vi "Polynomial Evaluation.vi"   [LabVIEW 2017, in "NI_AALPro.lvlib"]
doc: "Evaluates the polynomial <B>P(x)</B> with a single value or multiple values. The data types you wire to the <B>a</B> and <B>P(x)</B> inputs determine the polymorphic instance to use."
uses:
  <vilib>/Analysis/NI_AALPro.lvlib
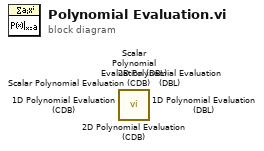
[diagram p0: block diagram]
diagram:
  n1 = call <vilib>:"2D Polynomial Evaluation (CDB).vi"() -> ()  [unwired: 2 in, 2 out]
  n2 = call <vilib>:"2D Polynomial Evaluation (DBL).vi"() -> ()  [unwired: 2 in, 2 out]
  n3 = call <vilib>:"1D Polynomial Evaluation (CDB).vi"() -> ()  [unwired: 2 in, 2 out]
  n4 = call <vilib>:"1D Polynomial Evaluation (DBL).vi"() -> ()  [unwired: 2 in, 2 out]
  n5 = call <vilib>:"Scalar Polynomial Evaluation (CDB).vi"() -> ()  [unwired: 2 in, 2 out]
  n6 = call <vilib>:"Scalar Polynomial Evaluation (DBL).vi"() -> ()  [unwired: 2 in, 2 out]
